vi "Components.vi"() -> ()   [LabVIEW 2023, in "Main.lvlib" / "Main.lvclass"]
uses:
  Library/Main.lvclass
panel:
  in  "ManualButtons":string="ManualButtons"
  in  "ManualUI":string="ManualUI"
  in  "Debugger":string="Debugger"
  in  "FaultMonitor":string="FaultMonitor"
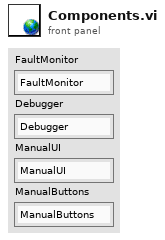
[diagram p1: front panel]
diagram:
